vi "In-Range (Greyscale).vi"(8 "error in (no error)":errorcluster, 9 "In-Range Image Colour Range":T1, 10 "In-Range-Result":T2, 11 "Greyscale Image-Source":T2) -> (0 "error out":errorcluster, 3 "In-Range-Result (duplicate)":T2)   [LabVIEW 2020, in "g_ar_toolkit.image.lvlib"]
uses:
  g_ar_toolkit.image.lvlib
  Greyscale Image.ctl
  In-Range Image Grey Range.ctl
  5701baee-35e2-4306-9a77-a9fdbb5b3a7f.vi
  g_ar_toolkit.common/Module Path.vi
  <vilib>/Utility/error.llb/Error Cluster From Error Code.vi
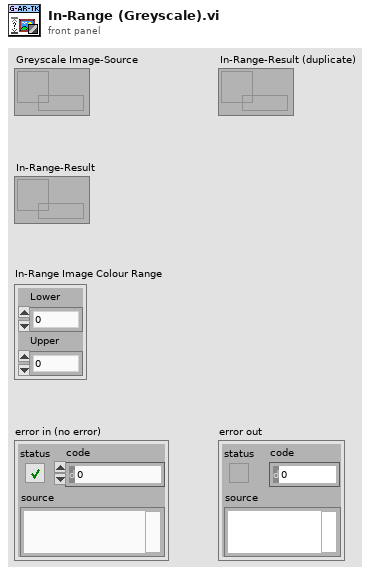
[diagram p1: front panel]
types:
  T1 = typedef "g_ar_toolkit.image.lvlib/In-Range Image Grey Range.ctl" = cluster{"Lower":u8, "Upper":u8}
  T2 = typedef "g_ar_toolkit.image.lvlib/Greyscale Image.ctl" = refnum<data-value>
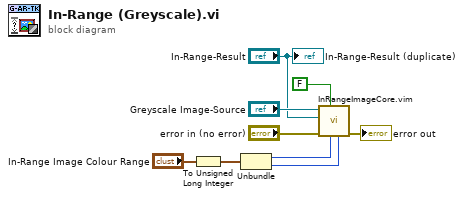
[diagram p0: block diagram]
diagram:
  n1 = To Unsigned Long Integer(number="In-Range Image Colour Range") -> (unsigned 32bit integer=w1:cluster{"Lower":u32, "Upper":u32})
  n2 = Unbundle(w1) -> ("Lower"=w4:u32, "Upper"=w8:u32)
  n3 = call "InRangeImageCore.vim"("Upper"=w8, "Lower"=w4, "IgnoreAlpha"=FALSE, "error in (no error)"="error in (no error)", "In-Range-Result"="In-Range-Result", "Src"="Greyscale Image-Source") -> ("error out"=→"error out":errorcluster)  [unwired: 5 in]
  "In-Range-Result (duplicate)" <- "In-Range-Result"
